vi "File & Folder.vi"(8 "error in (no error)":errorcluster) -> (0 "error out":errorcluster, 3 "Cluster":T1)   [LabVIEW 2022 SP3]
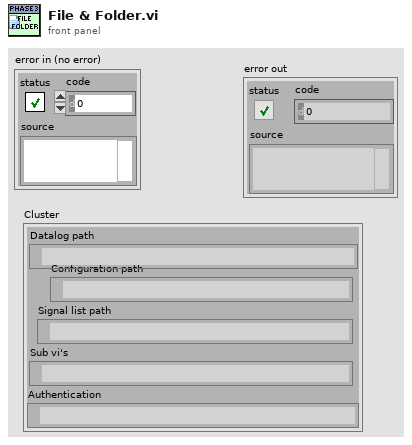
[diagram p1: front panel]
types:
  T1 = cluster{"Datalog path":path, "Configuration path":path, "Signal list path":path, "Sub vi's":path, "Authentication":path}
  T2 = enum32{"invalid app kind", "Development System", "Run Time System", "Student Edition", "Embedded LabVIEW", "Evaluation", "Custom"}
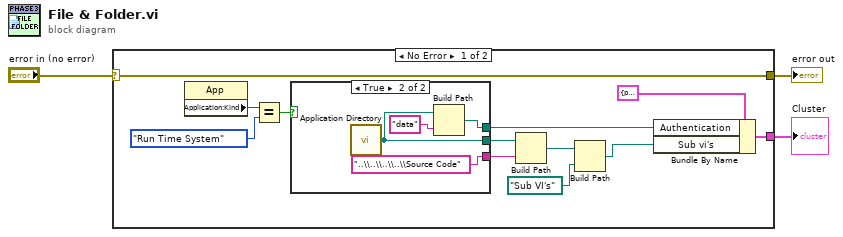
[diagram p0: block diagram]
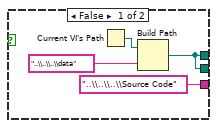
[diagram p2: hidden frame]
diagram:
  n1 = case shown="No Error" "error in (no error)" {
    selector: "error in (no error)" -> [w11 _]
    tunnel: [w11 _] -> w2
    tunnel: [w10 _] -> w1
    frame No Error {
      n2 = property class="App"() -> ("Application:Kind"=w15:T2)  [unwired: 2 in, 2 out]
      n3 = Equal?(x=w15, y=T2."Run Time System") -> (x = y?=w13:bool)
      n4 = case shown="True" w13 {
        tunnel: ["..\\..\\..\\Source Code" ("name or relative path") "..\\..\\..\\..\\Source Code" ("name or relative path")] -> w9
        tunnel: [w16 w22] -> w6
        tunnel: [w16 w21] -> w5
        frame False {
          n5 = Current VI's Path() -> (path=w17:path)
          n6 = Build Path(base path=w17, name or relative path="..\\..\\..\\data") -> (appended path=w16:path)
        }
        frame True {
          n7 = call <vilib>:"Application Directory.vi"() -> ("Application Directory"=w21:path)
          n8 = Build Path(base path=w21, name or relative path="data") -> (appended path=w22:path)
        }
      }
      n9 = Build Path(base path=w5, name or relative path=w9) -> (appended path=w8:path)
      n10 = Build Path(base path=w8, name or relative path=path "Sub VI's") -> (appended path=w4:path)
      n11 = Bundle By Name(cluster=T1 {"Datalog path"=path "", "Configuration path"=path "", "Signal list path"=path "", "Sub vi's"=path "", "Authentication"=path ""} ("Cluster"), "Authentication"=w6, "Sub vi's"=w4) -> (w10:T1)
    }
    frame Error {
    }
  }
  "error out" <- w2
  "Cluster" <- w1
